vi "StringPlayHouse.vi"() -> ()   [LabVIEW 2015]
uses:
  <vilib>/regexp/Match Regular Expression.xnode
panel:
  out "Array":T1(array[cluster])
  out "All Albums":string[](array[string])
  out "text 2":string="Amy Winehouse\nBack to Black\nRehab\t213\nYou Know I'm No Good\t257\nMe & Mr Jones\t152\nJust Friends\t192\nBack to Black\t240\nLove Is a Losing Game\t154\nTears Dry On Their Own\t185\nWake Up Alone\t221\nSome Unholy War\t141\nHe Can Only Hold Her\t166\nYou Know I'm No Good\t202\nRehab (Hot Chip Vocal)\t418\n\nThe Beach Boys\nPet Sounds [Bonus Tracks]\nWouldn't It Be Nice\t146\nYou Still Believe In Me\t155\nThat's Not Me\t150\nDon't Talk (Put Your Head On My Shoulder)\t174\nI'm Waiting For The Day\t186\nLet's Go Away For Awhile\t141\nSloop John B\t180\nGod Only Knows\t173\nI Know There's An Answer\t191\nHere Today\t175\nI Just Wasn't Made For These Times\t196\nPet Sounds\t143\nCaroline No\t174\nHang On To Your Ego\t184\n\nThe Beatles\nAbbey Road\nCome Together\t261\nSomething\t183\nMaxwell's Silver Hammer\t207\nOh! Darling\t207\nOctopus's Garden\t171\nI Want You (She's So Heavy)\t467\nHere Comes The Sun\t186\nBecause\t166\nYou Never Give Me Your Money\t242\nSun King\t146\nMean Mr. Mustard\t66\nPolythene Pam\t73\nShe Came In Through The Bathroom Window\t118\nGolden Slumbers\t92\nCarry That Weight\t97\nThe End\t140\nHer Majesty\t23\n\nBob Dylan\nNashville Skyline\nGirl From The North Country\t224\nNashville Skyline Rag\t195\nTo Be Alone With You\t131\nI Threw It All Away\t146\nPeggy Day\t125\nLay Lady Lay\t201\nOne More Night\t145\nTell Me That It Isn't True\t164\nCountry Pie\t99\nTonight I'll Be Staying Here With You\t203\n\nCAKE\nProlonging The Magic\nMexico\t206\nNever There\t164\nGuitar\t221\nYou Turn The Screws\t253\nWalk On By\t226\nSheep Go To Heaven\t285\nWhen You Sleep\t238\nHem Of Your Garment\t224\nAlpha Beta Parking Lot\t210\nLet Me Go\t236\nCool Blue Reason\t208\nWhere Would I Be?\t233\n\nChris Isaak\nHeart Shaped World\nHeart Shaped World\t210\nI'm Not Waiting\t196\nDon't Make Me Dream About You\t213\nKings Of The Highway\t287\nWicked Game\t289\nBlue Spanish Sky\t238\nWrong To Love You\t260\nForever Young\t203\nNothing's Changed\t248\nIn The Heat Of The Jungle\t380\nDiddley Daddy\t246\n\nChristina Aguilera\nStripped\nStripped Intro\t100\nCan't Hold Us Down\t256\nWalk Away\t347\nFighter\t246\nPrimer Amor\t54\nInfatuation\t258\nLoves Embrace\t47\nLoving Me 4 Me\t277\nImpossible\t254\nUnderappreciated\t241\nBeautiful\t239\nMake Over\t253\nCruz\t230\nSoar\t285\nGet Mine, Get Yours\t225\nDirrty\t299\nStripped Part 2\t46\nThe Voice Within\t304\nI'm OK\t320\nKeep On Singin' My Song\t390\n\nCulture Club\nColour By Numbers\nKarma Chameleon\t253\nIt's A Miracle\t205\nBlack Money\t319\nChanging Every Day\t198\nThat's The Way (I'm Only Trying To Help You)\t167\nChurch Of The Poison Mind\t211\nMiss Me Blind\t270\nMister Man\t216\nStormkeeper\t170\nVictims\t293\n\nCyndi Lauper\nTrue Colors\nChange Of Heart\t265\nMaybe He'll Know\t267\nBoy Blue\t287\nTrue Colors\t228\nCalm Inside The Storm\t235\nWhat's Going On\t279\nIko Iko\t130\nThe Faraway Nearby\t180\n911\t196\nOne Track Mind\t222\n\nDepeche Mode\nViolator\nWorld In My Eyes\t266\nSweetest Perfection\t284\nPersonal Jesus\t296\nHalo\t270\nWaiting For The Night\t367\nEnjoy The Silence\t373\nPolicy Of Truth\t295\nBlue Dress\t342\nClean\t329\n\nEdie Brickell & The New Bohemians\nShooting Rubberbands At The Stars\nWhat I Am\t298\nLittle Miss S.\t220\nAir Of December\t360\nThe Wheel\t235\nLove Like We Do\t189\nCircle\t193\nBeat The Time\t178\nShe\t309\nNothing\t291\nNow\t365\nKeep Coming Back\t166\nI Do\t121\n\nFiona Apple\nTidal\nSleep To Dream\t250\nSullen Girl\t235\nShadowboxer\t324\nCriminal\t343\nSlow Like Honey\t358\nThe First Taste\t287\nNever Is A Promise\t355\nThe Child Is Gone\t255\nPale September\t351\nCarrion\t346\n\nThe Fugees\nThe Score\nRed Intro\t112\nHow Many Mics\t269\nReady Or Not\t227\nZealots\t261\nThe Beast\t337\nFu-Gee-La\t260\nFamily Business\t344\nKilling Me Softly\t299\nThe Score\t302\nThe Mask\t291\nCowboys\t324\nNo Woman, No Cry\t273\nManifest/Outro\t360\nFu-Gee-La (Refugee Camp Remix)\t264\nFu-Gee-La (Refugee Camp Global Mix)\t327\nMista Mista\t163\n\nGary Allan\nSmoke Rings In The Dark\nSmoke Rings In The Dark\t259\nRight Where I Need To Be\t182\nDon't Tell Momma\t237\nLovin' You Against My Will\t239\nSorry\t187\nCryin' For Nothing\t258\nBourbon Borderline\t168\nRunaway\t165\nLearning To Live With Me\t156\nCowboy Blues\t178\nI'm The One\t198\nGreenfields\t192\n\nGeorge Michael\nFaith\nFaith\t196\nFather Figure\t337\nI Want Your Sex (Parts 1&2)\t557\nOne More Try\t351\nHard Day\t288\nHand To Mouth\t276\nLook At Your Hands\t278\nMonkey\t306\nKissing A Fool\t276\nHard Day (Shep Pettibone Remix)\t390\nA Last Request (I Want Your Sex Part III)\t228\n\nGuns N' Roses\nAppetite For Destruction\nWelcome To The Jungle\t274\nIt's So Easy\t203\nNightrain\t268\nOut Ta Get Me\t264\nMr. Brownstone\t229\nParadise City\t406\nMy Michelle\t220\nThink About You\t232\nSweet Child O' Mine\t356\nYou're Crazy\t197\nAnything Goes\t206\nRocket Queen\t373\n\nLauryn Hill\nThe Miseducation Of Lauryn Hill\nIntro\t47\nLost Ones\t334\nEx-Factor\t327\nTo Zion\t369\nDoo Wop (That Thing)\t320\nSuperstar\t297\nFinal Hour\t256\nWhen It Hurts So Bad\t342\nI Used To Love Him\t340\nForgive Them Father\t315\nEvery Ghetto, Every City\t315\nNothing Even Matters\t351\nEverything Is Everything\t293\nMiseducation Of Lauryn Hill\t257\nCan't Take My Eyes Off Of You\t221\nTell Him\t281\n\nLily Allen\nAlright, Still\nSmile\t197\nKnock 'Em Out\t174\nLDN\t191\nEverythings Just Wonderful\t209\nNot Big\t197\nFriday Night\t187\nShame for You\t246\nLittlest Things\t182\nTake What You Take\t246\nFriend of Mine\t238\nAlfie\t165\nNan You're a Window Shopper\t178\nSmile Version Revisited (Mark Ronson Remix)\t193\n\nSublime\n40 Oz. To Freedom\nWaiting For My Ruca\t140\n40 Oz. To Freedom\t183\nSmoke Two Joints\t173\nWe're Only Gonna Die For Our Arrogance\t187\nDon't Push\t259\n54-46 That's My Number / Ball And Chain\t318\nBadfish\t185\nLet's Go Get Stoned\t213\nNew Thrash\t90\nScarlet Begonias\t212\nLive At E's\t189\nDJs\t198\nChica Me Tipo\t136\nRight Back\t169\nWhat Happened\t208\nNew Song\t194\nEbin\t212\nDate Rape\t218\nHope\t103\nKRS-One\t144\nRivers Of Babylon\t149\nThank You Dub\t263\n"
  in  "text":string="Amy Winehouse\nBack to Black\nRehab\t213\nYou Know I'm No Good\t257\nMe & Mr Jones\t152\nJust Friends\t192\nBack to Black\t240\nLove Is a Losing Game\t154\nTears Dry On Their Own\t185\nWake Up Alone\t221\nSome Unholy War\t141\nHe Can Only Hold Her\t166\nYou Know I'm No Good\t202\nRehab (Hot Chip Vocal)\t418\n\nThe Beach Boys\nPet Sounds [Bonus Tracks]\nWouldn't It Be Nice\t146\nYou Still Believe In Me\t155\nThat's Not Me\t150\nDon't Talk (Put Your Head On My Shoulder)\t174\nI'm Waiting For The Day\t186\nLet's Go Away For Awhile\t141\nSloop John B\t180\nGod Only Knows\t173\nI Know There's An Answer\t191\nHere Today\t175\nI Just Wasn't Made For These Times\t196\nPet Sounds\t143\nCaroline No\t174\nHang On To Your Ego\t184\n\nThe Beatles\nAbbey Road\nCome Together\t261\nSomething\t183\nMaxwell's Silver Hammer\t207\nOh! Darling\t207\nOctopus's Garden\t171\nI Want You (She's So Heavy)\t467\nHere Comes The Sun\t186\nBecause\t166\nYou Never Give Me Your Money\t242\nSun King\t146\nMean Mr. Mustard\t66\nPolythene Pam\t73\nShe Came In Through The Bathroom Window\t118\nGolden Slumbers\t92\nCarry That Weight\t97\nThe End\t140\nHer Majesty\t23\n\nBob Dylan\nNashville Skyline\nGirl From The North Country\t224\nNashville Skyline Rag\t195\nTo Be Alone With You\t131\nI Threw It All Away\t146\nPeggy Day\t125\nLay Lady Lay\t201\nOne More Night\t145\nTell Me That It Isn't True\t164\nCountry Pie\t99\nTonight I'll Be Staying Here With You\t203\n\nCAKE\nProlonging The Magic\nMexico\t206\nNever There\t164\nGuitar\t221\nYou Turn The Screws\t253\nWalk On By\t226\nSheep Go To Heaven\t285\nWhen You Sleep\t238\nHem Of Your Garment\t224\nAlpha Beta Parking Lot\t210\nLet Me Go\t236\nCool Blue Reason\t208\nWhere Would I Be?\t233\n\nChris Isaak\nHeart Shaped World\nHeart Shaped World\t210\nI'm Not Waiting\t196\nDon't Make Me Dream About You\t213\nKings Of The Highway\t287\nWicked Game\t289\nBlue Spanish Sky\t238\nWrong To Love You\t260\nForever Young\t203\nNothing's Changed\t248\nIn The Heat Of The Jungle\t380\nDiddley Daddy\t246\n\nChristina Aguilera\nStripped\nStripped Intro\t100\nCan't Hold Us Down\t256\nWalk Away\t347\nFighter\t246\nPrimer Amor\t54\nInfatuation\t258\nLoves Embrace\t47\nLoving Me 4 Me\t277\nImpossible\t254\nUnderappreciated\t241\nBeautiful\t239\nMake Over\t253\nCruz\t230\nSoar\t285\nGet Mine, Get Yours\t225\nDirrty\t299\nStripped Part 2\t46\nThe Voice Within\t304\nI'm OK\t320\nKeep On Singin' My Song\t390\n\nCulture Club\nColour By Numbers\nKarma Chameleon\t253\nIt's A Miracle\t205\nBlack Money\t319\nChanging Every Day\t198\nThat's The Way (I'm Only Trying To Help You)\t167\nChurch Of The Poison Mind\t211\nMiss Me Blind\t270\nMister Man\t216\nStormkeeper\t170\nVictims\t293\n\nCyndi Lauper\nTrue Colors\nChange Of Heart\t265\nMaybe He'll Know\t267\nBoy Blue\t287\nTrue Colors\t228\nCalm Inside The Storm\t235\nWhat's Going On\t279\nIko Iko\t130\nThe Faraway Nearby\t180\n911\t196\nOne Track Mind\t222\n\nDepeche Mode\nViolator\nWorld In My Eyes\t266\nSweetest Perfection\t284\nPersonal Jesus\t296\nHalo\t270\nWaiting For The Night\t367\nEnjoy The Silence\t373\nPolicy Of Truth\t295\nBlue Dress\t342\nClean\t329\n\nEdie Brickell & The New Bohemians\nShooting Rubberbands At The Stars\nWhat I Am\t298\nLittle Miss S.\t220\nAir Of December\t360\nThe Wheel\t235\nLove Like We Do\t189\nCircle\t193\nBeat The Time\t178\nShe\t309\nNothing\t291\nNow\t365\nKeep Coming Back\t166\nI Do\t121\n\nFiona Apple\nTidal\nSleep To Dream\t250\nSullen Girl\t235\nShadowboxer\t324\nCriminal\t343\nSlow Like Honey\t358\nThe First Taste\t287\nNever Is A Promise\t355\nThe Child Is Gone\t255\nPale September\t351\nCarrion\t346\n\nThe Fugees\nThe Score\nRed Intro\t112\nHow Many Mics\t269\nReady Or Not\t227\nZealots\t261\nThe Beast\t337\nFu-Gee-La\t260\nFamily Business\t344\nKilling Me Softly\t299\nThe Score\t302\nThe Mask\t291\nCowboys\t324\nNo Woman, No Cry\t273\nManifest/Outro\t360\nFu-Gee-La (Refugee Camp Remix)\t264\nFu-Gee-La (Refugee Camp Global Mix)\t327\nMista Mista\t163\n\nGary Allan\nSmoke Rings In The Dark\nSmoke Rings In The Dark\t259\nRight Where I Need To Be\t182\nDon't Tell Momma\t237\nLovin' You Against My Will\t239\nSorry\t187\nCryin' For Nothing\t258\nBourbon Borderline\t168\nRunaway\t165\nLearning To Live With Me\t156\nCowboy Blues\t178\nI'm The One\t198\nGreenfields\t192\n\nGeorge Michael\nFaith\nFaith\t196\nFather Figure\t337\nI Want Your Sex (Parts 1&2)\t557\nOne More Try\t351\nHard Day\t288\nHand To Mouth\t276\nLook At Your Hands\t278\nMonkey\t306\nKissing A Fool\t276\nHard Day (Shep Pettibone Remix)\t390\nA Last Request (I Want Your Sex Part III)\t228\n\nGuns N' Roses\nAppetite For Destruction\nWelcome To The Jungle\t274\nIt's So Easy\t203\nNightrain\t268\nOut Ta Get Me\t264\nMr. Brownstone\t229\nParadise City\t406\nMy Michelle\t220\nThink About You\t232\nSweet Child O' Mine\t356\nYou're Crazy\t197\nAnything Goes\t206\nRocket Queen\t373\n\nLauryn Hill\nThe Miseducation Of Lauryn Hill\nIntro\t47\nLost Ones\t334\nEx-Factor\t327\nTo Zion\t369\nDoo Wop (That Thing)\t320\nSuperstar\t297\nFinal Hour\t256\nWhen It Hurts So Bad\t342\nI Used To Love Him\t340\nForgive Them Father\t315\nEvery Ghetto, Every City\t315\nNothing Even Matters\t351\nEverything Is Everything\t293\nMiseducation Of Lauryn Hill\t257\nCan't Take My Eyes Off Of You\t221\nTell Him\t281\n\nLily Allen\nAlright, Still\nSmile\t197\nKnock 'Em Out\t174\nLDN\t191\nEverythings Just Wonderful\t209\nNot Big\t197\nFriday Night\t187\nShame for You\t246\nLittlest Things\t182\nTake What You Take\t246\nFriend of Mine\t238\nAlfie\t165\nNan You're a Window Shopper\t178\nSmile Version Revisited (Mark Ronson Remix)\t193\n\nSublime\n40 Oz. To Freedom\nWaiting For My Ruca\t140\n40 Oz. To Freedom\t183\nSmoke Two Joints\t173\nWe're Only Gonna Die For Our Arrogance\t187\nDon't Push\t259\n54-46 That's My Number / Ball And Chain\t318\nBadfish\t185\nLet's Go Get Stoned\t213\nNew Thrash\t90\nScarlet Begonias\t212\nLive At E's\t189\nDJs\t198\nChica Me Tipo\t136\nRight Back\t169\nWhat Happened\t208\nNew Song\t194\nEbin\t212\nDate Rape\t218\nHope\t103\nKRS-One\t144\nRivers Of Babylon\t149\nThank You Dub\t263\n"
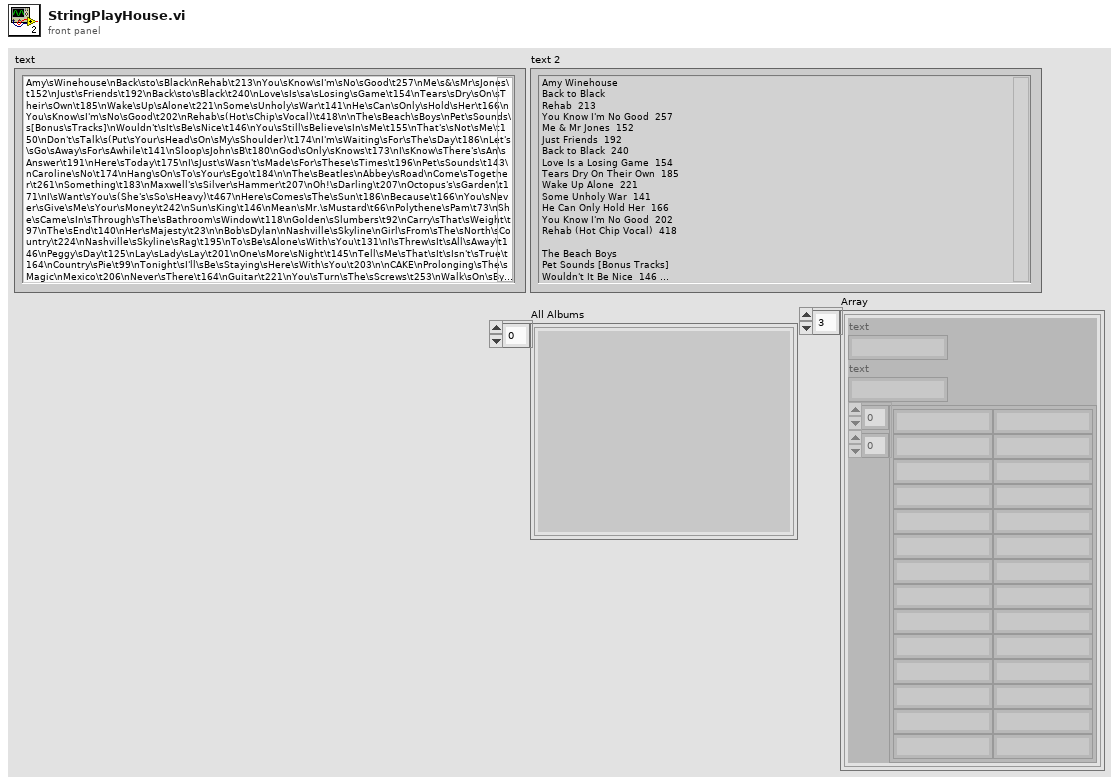
[diagram p1: front panel]
types:
  T1 = cluster{"text":string, "text":string, string[][]}[]
  T2 = cluster{"text":string, "text":string, string[][]}
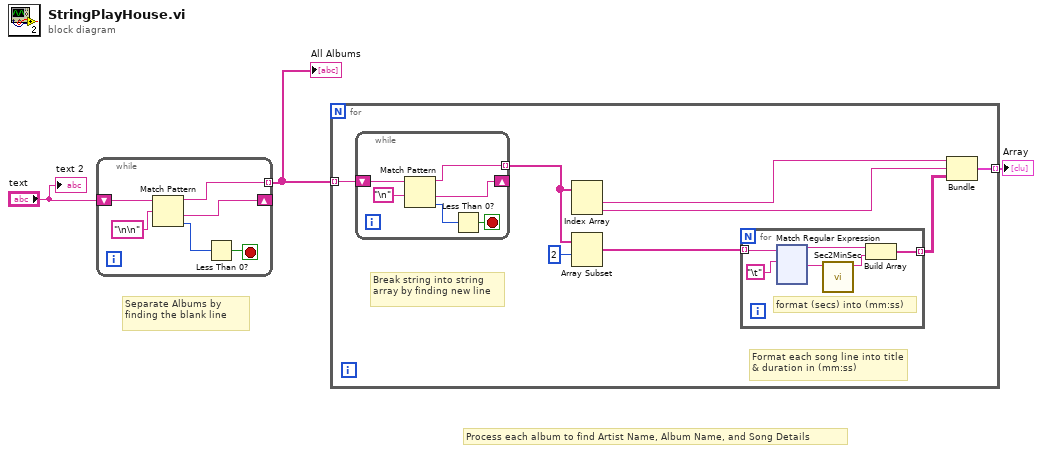
[diagram p0: block diagram]
diagram:
  # "Process each album to find Artist Name, Album Name, and Song Details"
  # "Separate Albums by finding the blank line"
  n1 = while {
    shift-right: [w5] -> _
    shift-left: "text" -> [w9]
    tunnel: [w4] -> w2 mode=indexing
    stop <- w6 stop-if-true
    n2 = Match Pattern(string=w9, regular expression="\n\n") -> (before substring=w4:string, after substring=w5:string, offset past match=w7:i32)  [unwired: 1 in, 1 out]
    n3 = Less Than 0?(x=w7) -> (x < 0?=w6:bool)
  }
  "All Albums" <- w2
  n4 = for {
    tunnel: w2 -> [w15] mode=indexing
    tunnel: [w10] -> w1 mode=indexing
    # "Format each song line into title & duration in (mm:ss)"
    # "Break string into string array by finding new line"
    n5 = while {
      shift-right: [w140] -> _
      shift-left: w15 -> [w141]
      tunnel: [w139] -> w17 mode=indexing
      stop <- w142 stop-if-true
      n6 = Match Pattern(string=w141, regular expression="\n") -> (before substring=w139:string, after substring=w140:string, offset past match=w143:i32)  [unwired: 1 in, 1 out]
      n7 = Less Than 0?(x=w143) -> (x < 0?=w142:bool)
    }
    n8 = Index Array "Index Array"(array=w17) -> (element #1=w13:string, element #2=w12:string)  [unwired: 2 in]
    n9 = Array Subset "Array Subset"(array=w17, index=2) -> (w14:string[])  [unwired: 1 in]
    n10 = for {
      tunnel: w14 -> [w23] mode=indexing
      tunnel: [w20] -> w11 mode=indexing
      # "format (secs) into (mm:ss)"
      n11 = xnode "Match Regular Expression"("input string"=w23, "regular expression"="\t") -> ("before match"=w22:string, "after match"=w19:string)  [unwired: 4 in, 3 out]
      n12 = call "Sec2MinSec.vi"("duration (s)"=w19) -> ("duration (mm:ss)"=w18:string)  [unwired: 10 in]
      n13 = Build Array(w22, w18) -> (w20:string[])
    }
    n14 = Bundle("text"=w13, "text"=w12, w11) -> (w10:T2)  [unwired: 1 in]
  }
  "Array" <- w1
  "text 2" <- "text"
